vi "IRunnable Small.vi"() -> (0 "IRunnable":refnum<class "IRunnable.lvclass">)   [LabVIEW 2024, in "IRunnable.lvclass"]
uses:
  IRunnable.lvclass
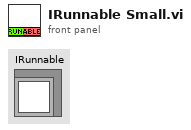
[diagram p1: front panel]
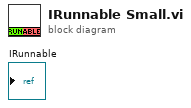
[diagram p0: block diagram]
diagram:
